vi "SoundSensor_Final.vi"() -> ()   [LabVIEW 2020]
uses:
  <vilib>/Analysis/baseanly.llb/Mean (DBL).vi
  <vilib>/Analysis/2dsp.llb/1D Auto Correlation (DBL).vi
  <vilib>/httpClient/PUTBuffer.vi
  <vilib>/express/express analysis/Spectral/Block/exnSpectralBlock spectral measurements peak poly.vi
  <vilib>/express/express analysis/Spectral/Block/exnSpectralBlock spectral measurements peak DDT.vi
  <vilib>/express/express analysis/Spectral/XNode/ExpressSpectralMeasurementsBlockNode.xnode
  <vilib>/Analysis/NI_AALBase.lvlib
  <vilib>/Analysis/NI_AALPro.lvlib
  <vilib>/httpClient/LabVIEWHTTPClient.lvlib
  <vilib>/ptbypt/NI_PtbyPt.lvlib
panel:
  out "BPM_Instant":dbl
  out "BPM_Mean":dbl
  out "BPM_3_Cycles":dbl
  out "Envelope fft sspectrum":dynamicdata(graph)
  out "low pass":dynamicdata(graph)
  out "After filtering 2":dynamicdata(graph)
  out "Before filtering 8000":dynamicdata(graph)
  in  "stop":bool
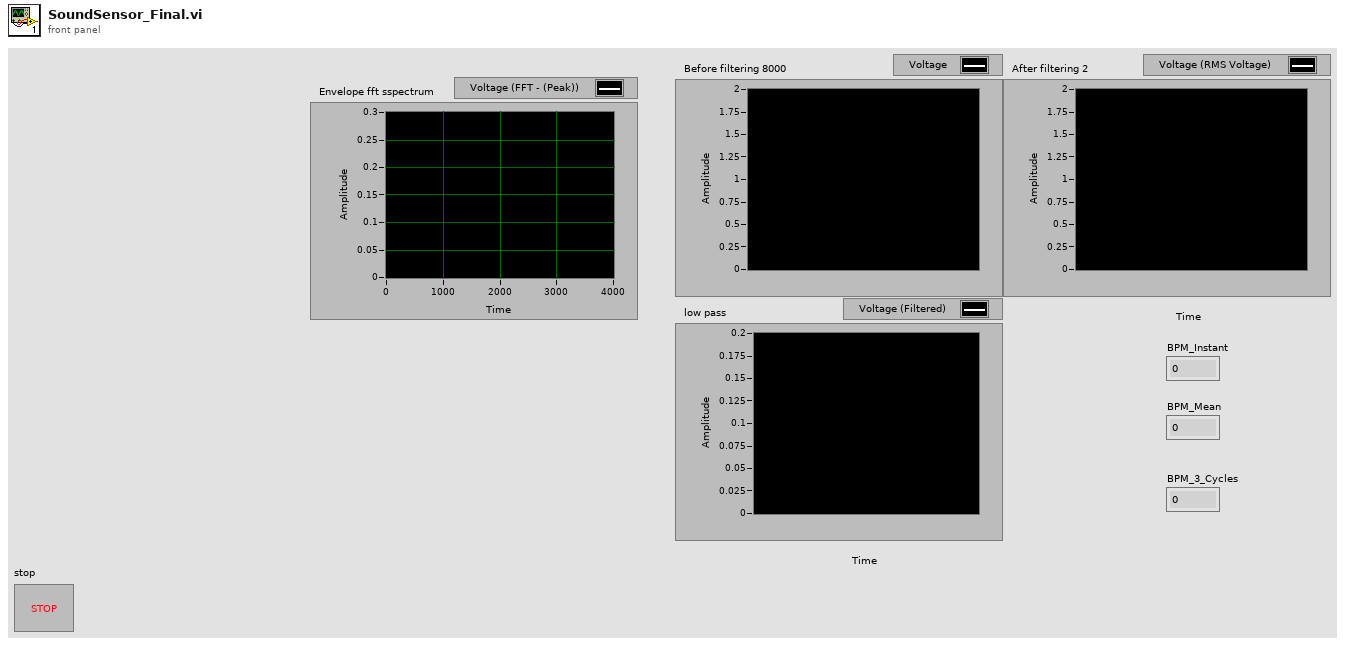
[diagram p1: front panel]
types:
  T1 = cluster{"averaging mode":u16, "weighting mode":u16, "number of averages":u32}
  T2 = cluster{"dB On (F)":bool, "unwrap phase (F)":bool, "convert to degree (F)":bool}
  T3 = typedef "LabVIEWHTTPClient.lvlib/ClientHandle.ctl" = refnum<k1>
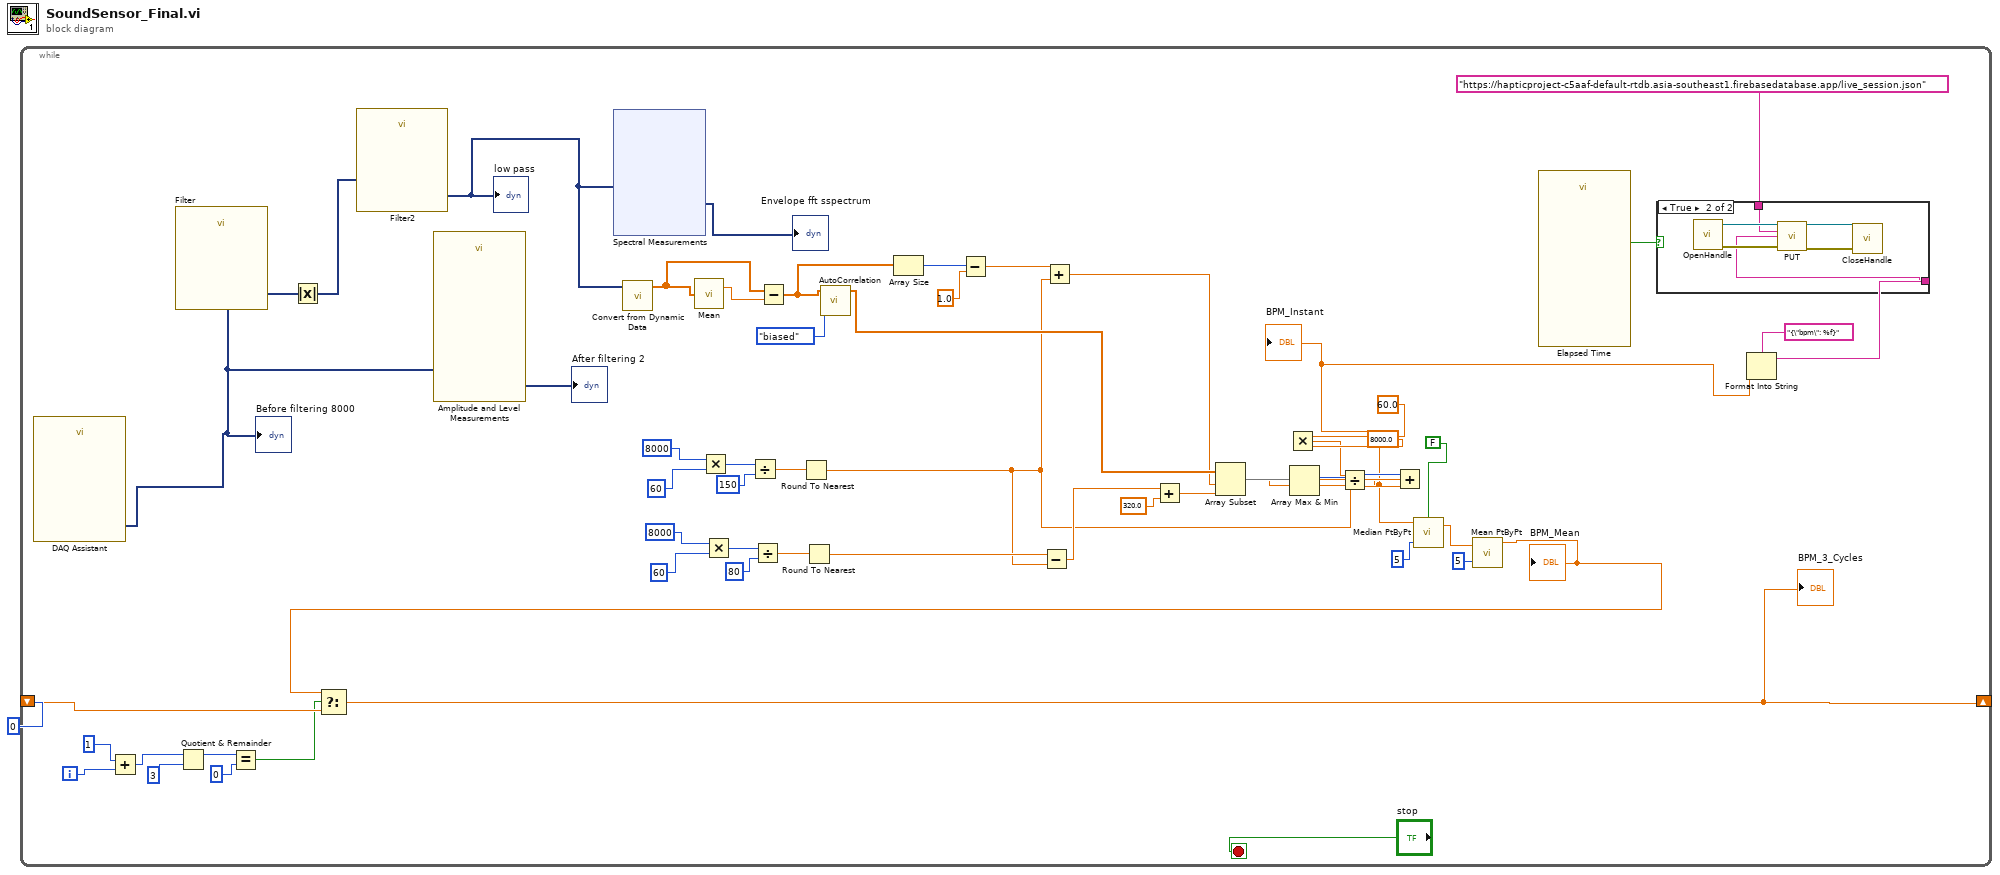
[diagram p0: block diagram]
diagram:
  n1 = while {
    shift-right: [w13] -> _
    shift-left: 0 -> [w15]
    i -> [w20]
    stop <- "stop" stop-if-true
    n2 = call "DAQ Assistant"() -> ("data"=w3:dynamicdata)  [unwired: 16 in, 3 out]
    "Before filtering 8000" <- w3
    n3 = Add(x=1, y=w20) -> (x+y=w19:i32)
    n4 = call "Filter"("Signal"=w3) -> ("Filtered Signal"=w55:dynamicdata)  [unwired: 9 in, 1 out]
    n5 = Quotient & Remainder(x=w19, y=3) -> (x-y*floor(x/y)=w17:i32)  [unwired: 1 out]
    n6 = Equal?(x=w17, y=0) -> (x = y?=w14:bool)
    n7 = Absolute Value(x=w55) -> (abs(x)=w54:dynamicdata)
    n8 = call "Filter2"("Signal"=w54) -> ("Filtered Signal"=w52:dynamicdata)  [unwired: 9 in, 1 out]
    "low pass" <- w52
    n9 = call "Amplitude and Level Measurements"("Signals"=w3) -> ("RMS"=→"After filtering 2":dynamicdata)  [unwired: 13 in, 1 out]
    n10 = xnode "Spectral Measurements"("Signals"=w52) -> ("FFT - (Peak)"=→"Envelope fft sspectrum":dynamicdata)  [unwired: 1 in, 2 out]
    n11 = call "Convert from Dynamic Data"("Dynamic Data Type"=w52) -> ("Array"=w51:dbl[])  [unwired: 3 in]
    n12 = call-poly <vilib>:"Mean.vi"("X"=w51) -> ("mean"=w50:dbl)  [unwired: 1 out]
    n13 = Multiply(x=8000, y=60) -> (x*y=w43:i32)
    n14 = Multiply(x=8000, y=60) -> (x*y=w39:i32)
    n15 = Divide(x=w43, y=150) -> (x/y=w42:dbl)
    n16 = Divide(x=w39, y=80) -> (x/y=w38:dbl)
    n17 = Subtract(x=w51, y=w50) -> (x-y=w48:dbl[])
    n18 = Round To Nearest(number=w42) -> (nearest integer value=w29:dbl)
    n19 = Round To Nearest(number=w38) -> (nearest integer value=w36:dbl)
    n20 = call-poly <vilib>:"AutoCorrelation.vi"("normalization"=enum32{"none", "unbiased", "biased"}."biased", "X"=w48) -> ("Rxx"=w34:dbl[])  [unwired: 8 in, 1 out]
    n21 = Array Size(array=w48) -> (size(s)=w46:i32)
    n22 = Subtract(x=w46, y=1.0) -> (x-y=w37:dbl)
    n23 = Subtract(x=w36, y=w29) -> (x-y=w35:dbl)
    n24 = Add(x=w37, y=w29) -> (x+y=w33:dbl)
    n25 = Add(x=w35, y=320.0) -> (x+y=w32:dbl)
    n26 = Array Subset(array=w34, index=w33, length=w32) -> (w31:dbl[])
    n27 = Multiply(x=60.0, y=8000.0) -> (x*y=w26:dbl)
    n28 = Array Max & Min(array=w31) -> (max index (indices)=w30:i32)  [unwired: 3 out]
    n29 = Add(x=w30, y=w29) -> (x+y=w25:dbl)
    n30 = Divide(x=w26, y=w25) -> (x/y=w2:dbl)
    "BPM_Instant" <- w2
    n31 = call <vilib>:"Median PtByPt.vi"("initialize"=FALSE, "sample length"=5, "x"=w2) -> ("median"=w6:dbl)  [unwired: 1 in, 1 out]
    n32 = call <vilib>:"Mean PtByPt.vi"("x"=w6, "sample length"=5) -> ("mean"=w5:dbl)  [unwired: 2 in, 1 out]
    "BPM_Mean" <- w5
    n33 = Select(t=w5, s=w14, f=w15) -> (s? t:f=w13:dbl)
    "BPM_3_Cycles" <- w13
    n34 = call "Elapsed Time"() -> ("Time has Elapsed"=w9:bool)  [unwired: 12 in, 7 out]
    n35 = Format Into String(format string="{\"bpm\": %f}", w2) -> (resulting string=w10:string)  [unwired: 2 in, 1 out]
    n36 = case shown="True" w9 {
      tunnel: "https://hapticproject-c5aaf-default-rtdb.asia-southeast1.firebasedatabase.app/live_session.json" ("url") -> [_ w59]
      tunnel: w10 -> [_ w58]
      frame False {
      }
      frame True {
        n37 = call <vilib>:"OpenHandle.vi"() -> ("client handle out"=w63:T3, "error out"=w61:errorcluster)  [unwired: 14 in]
        n38 = call-poly <vilib>:"PUT.vi"("client handle"=w63, "url"=w59, "buffer"=w58, "error in (no error)"=w61) -> ("client handle out"=w62:T3, "error out"=w60:errorcluster)  [unwired: 8 in, 2 out]
        n39 = call <vilib>:"CloseHandle.vi"("client handle"=w62, "error in (no error)"=w60) -> ()  [unwired: 13 in, 1 out]
      }
    }
  }
